vi "Insert String.vi"(9 "Offset":refnum<class "Abs_Numeric.lvclass">, 10 "New String":refnum<class "Abs_Value.lvclass">, 11 "String":refnum<class "Abs_String.lvclass">) -> (3 "Result":refnum<class "Abs_String.lvclass">)   [LabVIEW 2021]
uses:
  Abs_Types/String/Abs_String.lvclass
  Abs_Types/Value/Abs_Value.lvclass
  Abs_Types/Numeric/Abs_Numeric.lvclass
  Support/Insert/Insert_STR.lvclass
  C:/Program Files (x86)/National Instruments/LabVIEW 2021/vi.lib/TSA/Abstract Data Classes/Abs_Types/String/Abs_String.lvclass
  Support/Insert/Insert_STR.lvclass/Insert_STR.ctl
  Support/Insert/Properties/Write String.vi
  Support/Insert/Properties/Write Insert.vi
  Support/Insert/Properties/Write Offset.vi
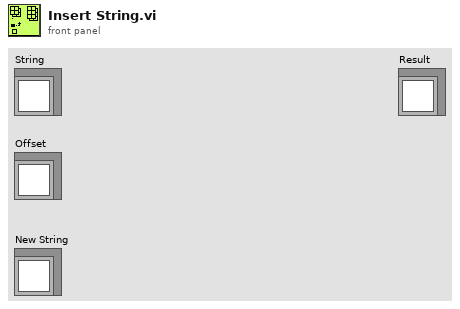
[diagram p1: front panel]
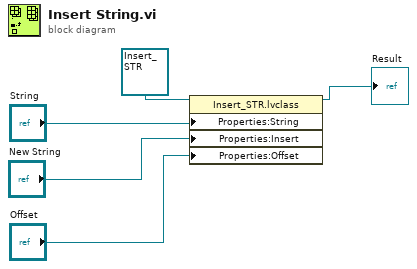
[diagram p0: block diagram]
diagram:
  n1 = property class="Insert_STR.lvclass"(reference=refnum<class "Insert_STR.lvclass"> refnum ("Insert_STR.lvclass"), "Properties:String"="String", "Properties:Insert"="New String", "Properties:Offset"="Offset") -> (reference out=→"Result":refnum<class "Insert_STR.lvclass">)  [unwired: 1 in, 1 out]
